vi "Convert ROI Type to Image Selection Tool.vi"(8 "Error In":errorcluster, 11 "ROI Type":u32(ring) items=["No Selection", "Point", "Line", "Rectangle", "Oval", "Polygon", "Freehand Region", "Annulus", "Unused2", "Unused3", "Broken Line", "Freehand Line", "Rotated Rectangle"]) -> (0 "Error Out":errorcluster, 3 "Image Selection Tool":T1 items=["Zoom Tool"=8, "Selection Tool"=0, "Pan Tool"=9, "Point Tool"=1, "Line Tool"=2, "Rectangle Tool"=3, "Rotated Rectangle Tool"=12, "Polyline Tool"=10, "Polygon Tool"=5, "Freehand Tool"=11, "Closed Freehand Tool"=6, "Ellipse Tool"=4, "Annulus Tool"=7])   [LabVIEW 2021, in "Image.lvlib"]
uses:
  Image.lvlib
  Image Selection Tool.ctl
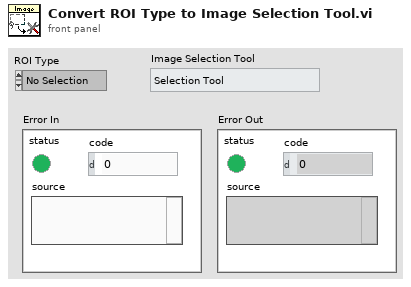
[diagram p1: front panel]
types:
  T1 = typedef "Image.lvlib/Image Selection Tool.ctl" = u32
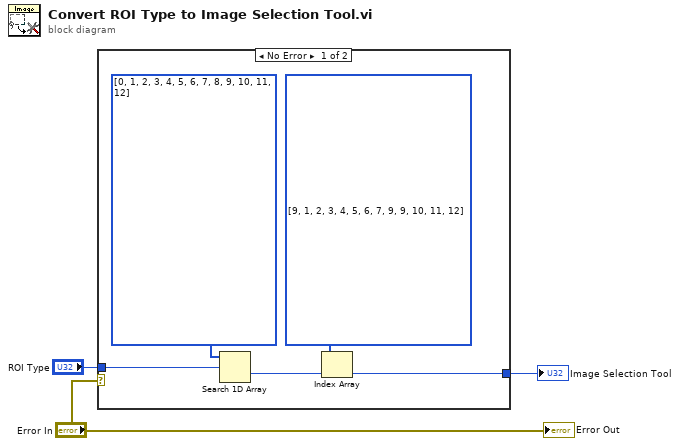
[diagram p0: block diagram]
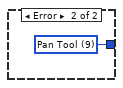
[diagram p2: hidden frame]
diagram:
  n1 = case shown="No Error" "Error In" {
    tunnel: "ROI Type" -> [w7 _]
    tunnel: [w4 w9] -> w2
    frame No Error {
      w6 = T1[] [9, 1, 2, 3, 4, 5, 6, 7, 9, 9, 10, 11, 12] items=["Zoom Tool"=8, "Selection Tool"=0, "Pan Tool"=9, "Point Tool"=1, "Line Tool"=2, "Rectangle Tool"=3, "Rotated Rectangle Tool"=12, "Polyline Tool"=10, "Polygon Tool"=5, "Freehand Tool"=11, "Closed Freehand Tool"=6, "Ellipse Tool"=4, "Annulus Tool"=7] ("Image Selection Tool")
      w8 = u32[] [0, 1, 2, 3, 4, 5, 6, 7, 8, 9, 10, 11, 12] items=["No Selection", "Point", "Line", "Rectangle", "Oval", "Polygon", "Freehand Region", "Annulus", "Unused2", "Unused3", "Broken Line", "Freehand Line", "Rotated Rectangle"] ("ROI Type")
      n2 = Search 1D Array(1D array=w8, element=w7) -> (index of element=w5:i32)  [unwired: 1 in]
      n3 = Index Array(array=w6, index=w5) -> (element=w4:T1)
    }
    frame Error {
      w9 = T1 9 items=["Zoom Tool"=8, "Selection Tool"=0, "Pan Tool"=9, "Point Tool"=1, "Line Tool"=2, "Rectangle Tool"=3, "Rotated Rectangle Tool"=12, "Polyline Tool"=10, "Polygon Tool"=5, "Freehand Tool"=11, "Closed Freehand Tool"=6, "Ellipse Tool"=4, "Annulus Tool"=7] ("Image Tool")
    }
  }
  "Image Selection Tool" <- w2
  "Error Out" <- "Error In"
